vi "Configure RF Power Ramp-Down.vi"(8 "error in (no error)":errorcluster, 10 "time, s":dbl, 11 "Comdel in":refnum<class "PL Comdel CX.lvclass">) -> (0 "error out":errorcluster, 3 "Comdel out":refnum<class "PL Comdel CX.lvclass">)   [LabVIEW 2015, in "PL Comdel CX.lvclass"]
doc: "Configures RF power ramp-down time. When disabled, RF power decreases to zero during specified <b>time</b>."
uses:
  PL Comdel CX.lvclass
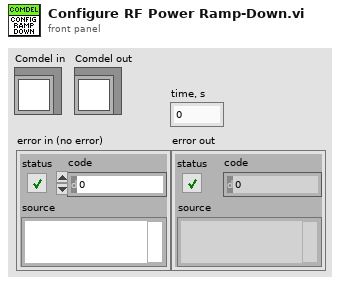
[diagram p1: front panel]
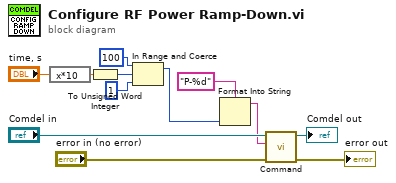
[diagram p0: block diagram]
diagram:
  n1 = expression code="x*10"("time, s") -> (w4:dbl)
  n2 = To Unsigned Word Integer(number=w4) -> (unsigned 16bit integer=w3:u16)
  n3 = In Range and Coerce(upper limit=u16 100, x=w3, lower limit=u16 1) -> (coerced(x)=w5:u16)  [unwired: 1 out]
  n4 = Format Into String(format string="P-%d", w5) -> (resulting string=w7:string)  [unwired: 2 in, 1 out]
  n5 = call "Command.vi"("error in (no error)"="error in (no error)", "command"=w7, "Comdel in"="Comdel in") -> ("error out"=→"error out":errorcluster, "Comdel out"=→"Comdel out":refnum<class "PL Comdel CX.lvclass">)  [unwired: 6 in, 1 out]
